vi "slider driver -- real.vi"(0 "slider in":refnum<vi>, 1 "slider action":T1, 9 "slider from":refnum<vi>, 11 "value IN":dbl=5700.934579439253, 12 "default":dbl=5700.934579439253) -> (4 "slider out":refnum<vi>, 6 "max":dbl, 8 "rel OUT":dbl, 10 "min":dbl, 15 "value OUT":dbl=5700.934579439253)   [LabVIEW 2018]
uses:
  slider action.ctl
  Q - not nan -- real.vi
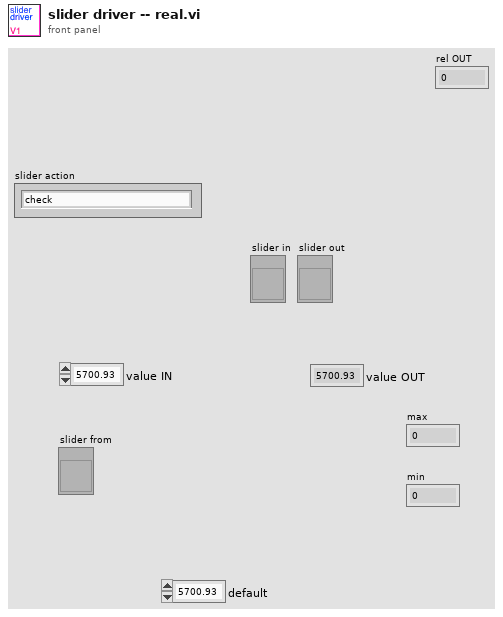
[diagram p1: front panel]
types:
  T1 = typedef "slider action.ctl" = enum16{"check", "copy range -- keep value", "set from value", "set from ratio", "set from slider", "read using other slider", "set lower limit", "set upper limit", "set lower from slider", "set upper from slider", "copy range -- keep ratio", "set using other slider -- no check"}
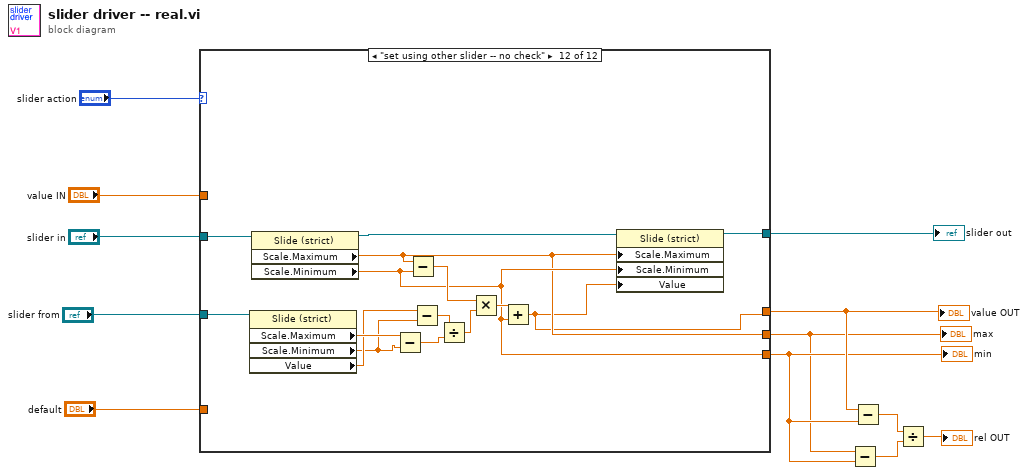
[diagram p0: block diagram]
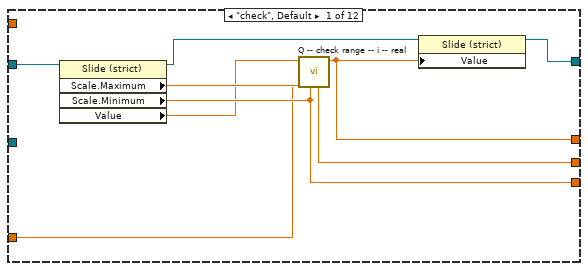
[diagram p2: hidden frame]
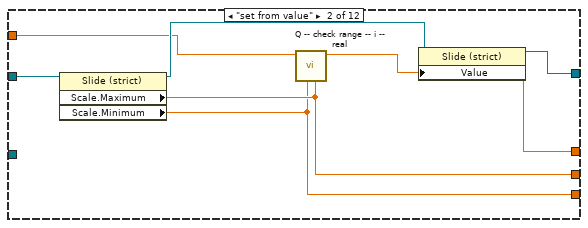
[diagram p3: hidden frame]
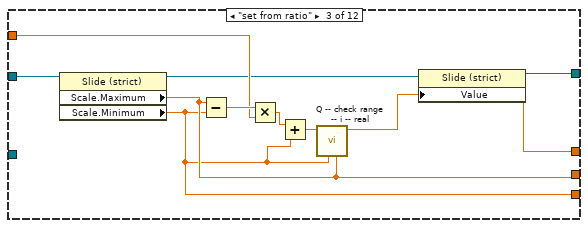
[diagram p4: hidden frame]
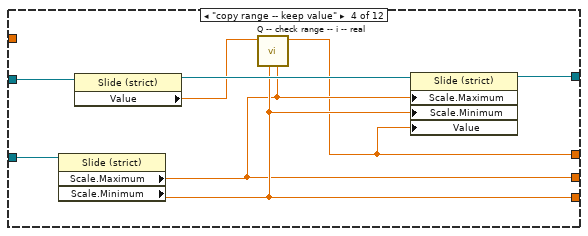
[diagram p5: hidden frame]
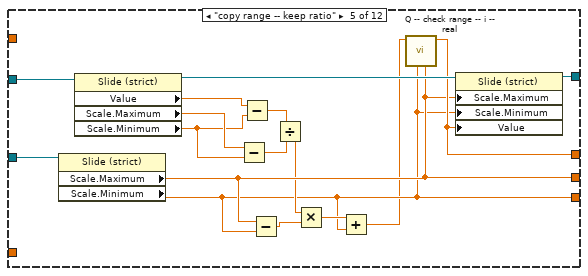
[diagram p6: hidden frame]
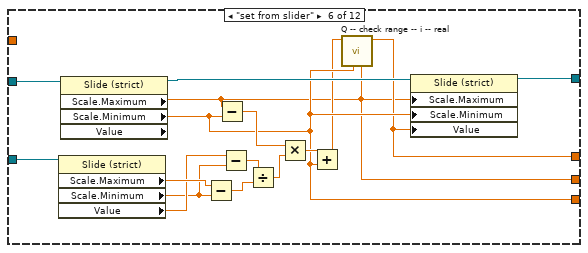
[diagram p7: hidden frame]
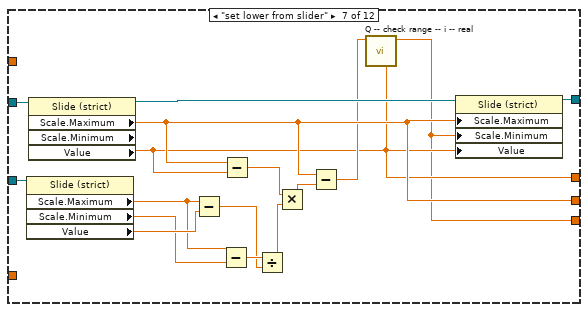
[diagram p8: hidden frame]
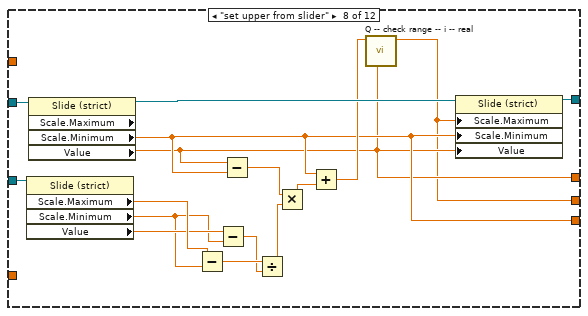
[diagram p9: hidden frame]
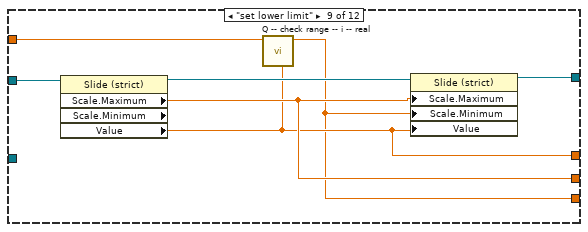
[diagram p10: hidden frame]
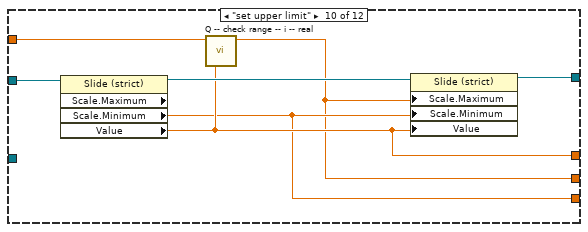
[diagram p11: hidden frame]
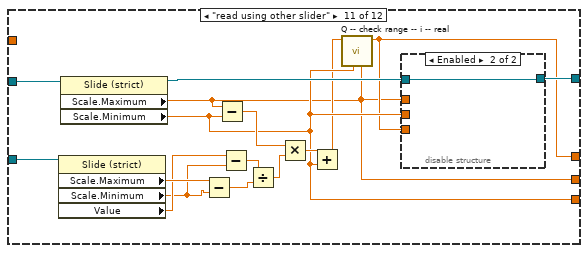
[diagram p12: hidden frame]
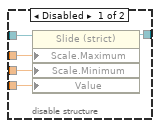
[diagram p13: hidden frame]
diagram:
  n1 = case shown="\"set using other slider -- no check\"" "slider action" {
    tunnel: "slider in" -> [w20 w27 w37 w43 w59 w75 w91 w107 w115 w122 w137 w158]
    tunnel: [w19 w26 w36 w38 w57 w63 w79 w95 w111 w119 w125 w146] -> w6
    tunnel: [w17 w24 w35 w44 w60 w76 w92 w108 w116 w123 w138 w159] -> w2
    tunnel: "slider from" -> [_ _ _ w45 w61 w77 w93 w109 _ _ w139 w160]
    tunnel: [w15 w22 w30 w40 w47 w65 w78 w96 w110 w118 w127 w148] -> w5
    tunnel: [w16 w23 w34 w39 w51 w62 w82 w94 w113 w117 w124 w147] -> w4
    tunnel: "value IN" -> [_ w21 w32 _ _ _ _ _ w114 w121 _ _]
    tunnel: "default" -> [w14 _ _ _ _ _ _ _ _ _ _ _]
    frame "check", Default {
      n2 = property class="Slide (strict)"(reference=w20) -> (reference out=w18:refnum<vi>, "Scale.Maximum"=w16:dbl, "Scale.Minimum"=w15:dbl, "Value"=w13:dbl)  [unwired: 1 in, 1 out]
      n3 = call "Q -- check range -- i -- real.vi"("upper"=w16, "lower"=w15, "default"=w14, "number"=w13) -> ("number in range"=w19:dbl)  [unwired: 5 in, 2 out]
      n4 = property class="Slide (strict)"(reference=w18, "Value"=w19) -> (reference out=w17:refnum<vi>)  [unwired: 1 in, 1 out]
    }
    frame "set from value" {
      n5 = property class="Slide (strict)"(reference=w27) -> (reference out=w25:refnum<vi>, "Scale.Maximum"=w23:dbl, "Scale.Minimum"=w22:dbl)  [unwired: 1 in, 1 out]
      n6 = call "Q -- check range -- i -- real.vi"("upper"=w23, "lower"=w22, "number"=w21) -> ("number in range"=w26:dbl)  [unwired: 6 in, 2 out]
      n7 = property class="Slide (strict)"(reference=w25, "Value"=w26) -> (reference out=w24:refnum<vi>)  [unwired: 1 in, 1 out]
    }
    frame "set from ratio" {
      n8 = property class="Slide (strict)"(reference=w37) -> (reference out=w31:refnum<vi>, "Scale.Maximum"=w34:dbl, "Scale.Minimum"=w30:dbl)  [unwired: 1 in, 1 out]
      n9 = Subtract(x=w34, y=w30) -> (x-y=w33:dbl)
      n10 = Multiply(x=w33, y=w32) -> (x*y=w29:dbl)
      n11 = Add(x=w29, y=w30) -> (x+y=w28:dbl)
      n12 = call "Q -- check range -- i -- real.vi"("upper"=w34, "lower"=w30, "number"=w28) -> ("number in range"=w36:dbl)  [unwired: 6 in, 2 out]
      n13 = property class="Slide (strict)"(reference=w31, "Value"=w36) -> (reference out=w35:refnum<vi>)  [unwired: 1 in, 1 out]
    }
    frame "copy range -- keep value" {
      n14 = property class="Slide (strict)"(reference=w45) -> ("Scale.Maximum"=w39:dbl, "Scale.Minimum"=w40:dbl)  [unwired: 1 in, 2 out]
      n15 = property class="Slide (strict)"(reference=w43) -> (reference out=w42:refnum<vi>, "Value"=w41:dbl)  [unwired: 1 in, 1 out]
      n16 = call "Q -- check range -- i -- real.vi"("upper"=w39, "lower"=w40, "number"=w41) -> ("number in range"=w38:dbl)  [unwired: 6 in, 2 out]
      n17 = property class="Slide (strict)"(reference=w42, "Scale.Maximum"=w39, "Scale.Minimum"=w40, "Value"=w38) -> (reference out=w44:refnum<vi>)  [unwired: 1 in, 1 out]
    }
    frame "copy range -- keep ratio" {
      n18 = property class="Slide (strict)"(reference=w61) -> ("Scale.Maximum"=w51:dbl, "Scale.Minimum"=w47:dbl)  [unwired: 1 in, 2 out]
      n19 = property class="Slide (strict)"(reference=w59) -> (reference out=w58:refnum<vi>, "Value"=w54:dbl, "Scale.Maximum"=w53:dbl, "Scale.Minimum"=w52:dbl)  [unwired: 1 in, 1 out]
      n20 = Subtract(x=w53, y=w52) -> (x-y=w55:dbl)
      n21 = Subtract(x=w54, y=w52) -> (x-y=w56:dbl)
      n22 = Subtract(x=w51, y=w47) -> (x-y=w49:dbl)
      n23 = Divide(x=w56, y=w55) -> (x/y=w50:dbl)
      n24 = Multiply(x=w50, y=w49) -> (x*y=w48:dbl)
      n25 = Add(x=w48, y=w47) -> (x+y=w46:dbl)
      n26 = call "Q -- check range -- i -- real.vi"("upper"=w51, "lower"=w47, "number"=w46) -> ("number in range"=w57:dbl)  [unwired: 6 in, 2 out]
      n27 = property class="Slide (strict)"(reference=w58, "Scale.Maximum"=w51, "Scale.Minimum"=w47, "Value"=w57) -> (reference out=w60:refnum<vi>)  [unwired: 1 in, 1 out]
    }
    frame "set from slider" {
      n28 = property class="Slide (strict)"(reference=w77) -> ("Scale.Maximum"=w73:dbl, "Scale.Minimum"=w71:dbl, "Value"=w72:dbl)  [unwired: 1 in, 2 out]
      n29 = property class="Slide (strict)" props=["Scale", "Maximum", "Scale", "Minimum", "Value"](reference=w75) -> (reference out=w74:refnum<vi>, "Scale.Maximum"=w62:dbl, "Scale.Minimum"=w65:dbl)  [unwired: 1 in, 2 out]
      n30 = Subtract(x=w73, y=w71) -> (x-y=w69:dbl)
      n31 = Subtract(x=w62, y=w65) -> (x-y=w67:dbl)
      n32 = Subtract(x=w72, y=w71) -> (x-y=w70:dbl)
      n33 = Divide(x=w70, y=w69) -> (x/y=w68:dbl)
      n34 = Multiply(x=w67, y=w68) -> (x*y=w66:dbl)
      n35 = Add(x=w66, y=w65) -> (x+y=w64:dbl)
      n36 = call "Q -- check range -- i -- real.vi"("upper"=w62, "lower"=w65, "number"=w64) -> ("number in range"=w63:dbl)  [unwired: 6 in, 2 out]
      n37 = property class="Slide (strict)"(reference=w74, "Scale.Maximum"=w62, "Scale.Minimum"=w65, "Value"=w63) -> (reference out=w76:refnum<vi>)  [unwired: 1 in, 1 out]
    }
    frame "set lower from slider" {
      n38 = property class="Slide (strict)"(reference=w93) -> ("Scale.Maximum"=w87:dbl, "Scale.Minimum"=w86:dbl, "Value"=w88:dbl)  [unwired: 1 in, 2 out]
      n39 = property class="Slide (strict)" props=["Scale", "Maximum", "Scale", "Minimum", "Value"](reference=w91) -> (reference out=w90:refnum<vi>, "Scale.Maximum"=w82:dbl, "Value"=w79:dbl)  [unwired: 1 in, 2 out]
      n40 = Subtract(x=w87, y=w88) -> (x-y=w85:dbl)
      n41 = Subtract(x=w87, y=w86) -> (x-y=w89:dbl)
      n42 = Subtract(x=w82, y=w79) -> (x-y=w84:dbl)
      n43 = Divide(x=w89, y=w85) -> (x/y=w83:dbl)
      n44 = Multiply(x=w84, y=w83) -> (x*y=w81:dbl)
      n45 = Subtract(x=w82, y=w81) -> (x-y=w80:dbl)
      n46 = call "Q -- check range -- i -- real.vi"("upper"=w79, "number"=w80) -> ("number in range"=w78:dbl)  [unwired: 7 in, 2 out]
      n47 = property class="Slide (strict)"(reference=w90, "Scale.Maximum"=w82, "Scale.Minimum"=w78, "Value"=w79) -> (reference out=w92:refnum<vi>)  [unwired: 1 in, 1 out]
    }
    frame "set upper from slider" {
      n48 = property class="Slide (strict)"(reference=w109) -> ("Scale.Maximum"=w104:dbl, "Scale.Minimum"=w97:dbl, "Value"=w98:dbl)  [unwired: 1 in, 2 out]
      n49 = property class="Slide (strict)" props=["Scale", "Maximum", "Scale", "Minimum", "Value"](reference=w107) -> (reference out=w106:refnum<vi>, "Scale.Minimum"=w96:dbl, "Value"=w95:dbl)  [unwired: 1 in, 2 out]
      n50 = Subtract(x=w104, y=w97) -> (x-y=w105:dbl)
      n51 = Subtract(x=w98, y=w97) -> (x-y=w103:dbl)
      n52 = Subtract(x=w95, y=w96) -> (x-y=w102:dbl)
      n53 = Divide(x=w105, y=w103) -> (x/y=w101:dbl)
      n54 = Multiply(x=w102, y=w101) -> (x*y=w100:dbl)
      n55 = Add(x=w96, y=w100) -> (x+y=w99:dbl)
      n56 = call "Q -- check range -- i -- real.vi"("lower"=w95, "number"=w99) -> ("number in range"=w94:dbl)  [unwired: 7 in, 2 out]
      n57 = property class="Slide (strict)"(reference=w106, "Scale.Maximum"=w94, "Scale.Minimum"=w96, "Value"=w95) -> (reference out=w108:refnum<vi>)  [unwired: 1 in, 1 out]
    }
    frame "set lower limit" {
      n58 = property class="Slide (strict)" props=["Scale", "Maximum", "Scale", "Minimum", "Value"](reference=w115) -> (reference out=w112:refnum<vi>, "Scale.Maximum"=w113:dbl, "Value"=w111:dbl)  [unwired: 1 in, 2 out]
      n59 = call "Q -- check range -- i -- real.vi"("upper"=w111, "number"=w114) -> ("number in range"=w110:dbl)  [unwired: 7 in, 2 out]
      n60 = property class="Slide (strict)"(reference=w112, "Scale.Maximum"=w113, "Scale.Minimum"=w110, "Value"=w111) -> (reference out=w116:refnum<vi>)  [unwired: 1 in, 1 out]
    }
    frame "set upper limit" {
      n61 = property class="Slide (strict)" props=["Scale", "Maximum", "Scale", "Minimum", "Value"](reference=w122) -> (reference out=w120:refnum<vi>, "Scale.Minimum"=w118:dbl, "Value"=w119:dbl)  [unwired: 1 in, 2 out]
      n62 = call "Q -- check range -- i -- real.vi"("lower"=w119, "number"=w121) -> ("number in range"=w117:dbl)  [unwired: 7 in, 2 out]
      n63 = property class="Slide (strict)"(reference=w120, "Scale.Maximum"=w117, "Scale.Minimum"=w118, "Value"=w119) -> (reference out=w123:refnum<vi>)  [unwired: 1 in, 1 out]
    }
    frame "read using other slider" {
      n64 = property class="Slide (strict)"(reference=w139) -> ("Scale.Maximum"=w135:dbl, "Scale.Minimum"=w133:dbl, "Value"=w134:dbl)  [unwired: 1 in, 2 out]
      n65 = property class="Slide (strict)"(reference=w137) -> (reference out=w136:refnum<vi>, "Scale.Maximum"=w124:dbl, "Scale.Minimum"=w127:dbl)  [unwired: 1 in, 1 out]
      n66 = Subtract(x=w135, y=w133) -> (x-y=w131:dbl)
      n67 = Subtract(x=w124, y=w127) -> (x-y=w129:dbl)
      n68 = Subtract(x=w134, y=w133) -> (x-y=w132:dbl)
      n69 = Divide(x=w132, y=w131) -> (x/y=w130:dbl)
      n70 = Multiply(x=w129, y=w130) -> (x*y=w128:dbl)
      n71 = Add(x=w128, y=w127) -> (x+y=w126:dbl)
      n72 = call "Q -- check range -- i -- real.vi"("upper"=w124, "lower"=w127, "number"=w126) -> ("number in range"=w125:dbl)  [unwired: 6 in, 2 out]
      n73 = disable-structure shown="Enabled" {
        disable-tunnel: [w144 w145] -> w138
        disable-tunnel: w136 -> [w143 w145]
        disable-tunnel: w127 -> [w142 _]
        disable-tunnel: w125 -> [w141 _]
        disable-tunnel: w124 -> [w140 _]
        frame Disabled {
          n74 = property class="Slide (strict)"(reference=w143, "Scale.Maximum"=w140, "Scale.Minimum"=w142, "Value"=w141) -> (reference out=w144:refnum<vi>)  [unwired: 1 in, 1 out]
        }
        frame Enabled {
        }
      }
    }
    frame "set using other slider -- no check" {
      n75 = property class="Slide (strict)"(reference=w160) -> ("Scale.Maximum"=w156:dbl, "Scale.Minimum"=w154:dbl, "Value"=w155:dbl)  [unwired: 1 in, 2 out]
      n76 = property class="Slide (strict)"(reference=w158) -> (reference out=w157:refnum<vi>, "Scale.Maximum"=w147:dbl, "Scale.Minimum"=w148:dbl)  [unwired: 1 in, 1 out]
      n77 = Subtract(x=w156, y=w154) -> (x-y=w152:dbl)
      n78 = Subtract(x=w147, y=w148) -> (x-y=w150:dbl)
      n79 = Subtract(x=w155, y=w154) -> (x-y=w153:dbl)
      n80 = Divide(x=w153, y=w152) -> (x/y=w151:dbl)
      n81 = Multiply(x=w150, y=w151) -> (x*y=w149:dbl)
      n82 = Add(x=w149, y=w148) -> (x+y=w146:dbl)
      n83 = property class="Slide (strict)"(reference=w157, "Scale.Maximum"=w147, "Scale.Minimum"=w148, "Value"=w146) -> (reference out=w159:refnum<vi>)  [unwired: 1 in, 1 out]
    }
  }
  "value OUT" <- w6
  "min" <- w5
  "max" <- w4
  "slider out" <- w2
  n84 = Subtract(x=w4, y=w5) -> (x-y=w7:dbl)
  n85 = Subtract(x=w6, y=w5) -> (x-y=w8:dbl)
  n86 = Divide(x=w8, y=w7) -> (x/y=→"rel OUT":dbl)
